vi "FlatToRichniswitch_grpc_ConfigureScanTriggerRequest.vi"(5 "OutputClusterType":T1, 11 "InputCluster":T3) -> (3 "OutputCluster":T1)   [LabVIEW 2021, in "NI Switch_client.lvlib"]
uses:
  NI Switch_client.lvlib
  niswitch_grpc_ConfigureScanTriggerRequest_trigger_input_enum/niswitch_grpc_ConfigureScanTriggerRequest_trigger_input_enum.lvclass
  niswitch_grpc_ConfigureScanTriggerRequest_scan_advanced_output_enum/niswitch_grpc_ConfigureScanTriggerRequest_scan_advanced_output_enum.lvclass
  nidevice_grpc_Session.ctl
  niswitch_grpc_ConfigureScanTriggerRequest.ctl
  niswitch_grpc_ScanAdvancedOutput.ctl
  niswitch_grpc_TriggerInput.ctl
  nidevice_grpc_Session_Flat.ctl
  niswitch_grpc_ConfigureScanTriggerRequest_Flat.ctl
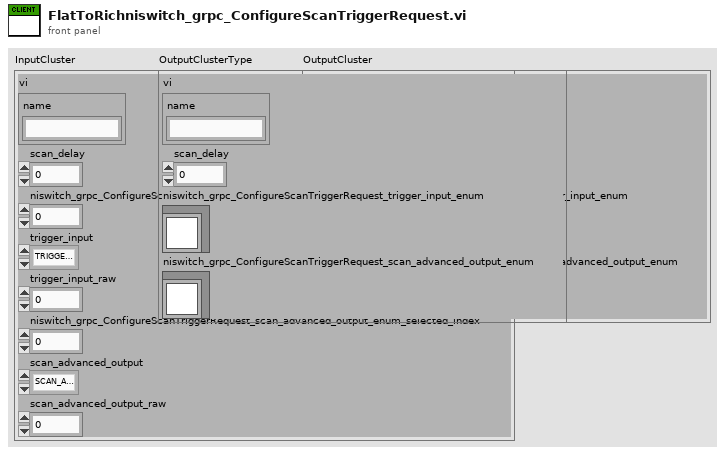
[diagram p1: front panel]
types:
  T1 = typedef "NI Switch_client.lvlib/niswitch_grpc_ConfigureScanTriggerRequest.ctl" = cluster{"vi":T2, "scan_delay":dbl, "niswitch_grpc_ConfigureScanTriggerRequest_trigger_input_enum":refnum<class "niswitch_grpc_ConfigureScanTriggerRequest_trigger_input_enum.lvclass">, "niswitch_grpc_ConfigureScanTriggerRequest_scan_advanced_output_enum":refnum<class "niswitch_grpc_ConfigureScanTriggerRequest_scan_advanced_output_enum.lvclass">}
  T2 = typedef "NI Switch_client.lvlib/nidevice_grpc_Session.ctl" = cluster{"name":string}
  T3 = typedef "NI Switch_client.lvlib/niswitch_grpc_ConfigureScanTriggerRequest_Flat.ctl" = cluster{"vi":T4, "scan_delay":dbl, "niswitch_grpc_ConfigureScanTriggerRequest_trigger_input_enum_selected_index":i32, "trigger_input":T5, "trigger_input_raw":i32, "niswitch_grpc_ConfigureScanTriggerRequest_scan_advanced_output_enum_selected_index":i32, "scan_advanced_output":T6, "scan_advanced_output_raw":i32}
  T4 = typedef "NI Switch_client.lvlib/nidevice_grpc_Session_Flat.ctl" = cluster{"name":string}
  T5 = typedef "NI Switch_client.lvlib/niswitch_grpc_TriggerInput.ctl" = enum32{"TRIGGER_INPUT_UNSPECIFIED", "TRIGGER_INPUT_NISWITCH_VAL_IMMEDIATE", "TRIGGER_INPUT_NISWITCH_VAL_EXTERNAL", "TRIGGER_INPUT_NISWITCH_VAL_SOFTWARE_TRIG", "TRIGGER_INPUT_NISWITCH_VAL_TTL0", "TRIGGER_INPUT_NISWITCH_VAL_TTL1", "TRIGGER_INPUT_NISWITCH_VAL_TTL2", "TRIGGER_INPUT_NISWITCH_VAL_TTL3", "TRIGGER_INPUT_NISWITCH_VAL_TTL4", "TRIGGER_INPUT_NISWITCH_VAL_TTL5", "TRIGGER_INPUT_NISWITCH_VAL_TTL6", "TRIGGER_INPUT_NISWITCH_VAL_TTL7", "TRIGGER_INPUT_NISWITCH_VAL_PXI_STAR", "TRIGGER_INPUT_NISWITCH_VAL_REARCONNECTOR", "TRIGGER_INPUT_NISWITCH_VAL_FRONTCONNECTOR", "TRIGGER_INPUT_NISWITCH_VAL_REARCONNECTOR_MODULE1", "TRIGGER_INPUT_NISWITCH_VAL_REARCONNECTOR_MODULE2", "TRIGGER_INPUT_NISWITCH_VAL_REARCONNECTOR_MODULE3", "TRIGGER_INPUT_NISWITCH_VAL_REARCONNECTOR_MODULE4", "TRIGGER_INPUT_NISWITCH_VAL_REARCONNECTOR_MODULE5", "TRIGGER_INPUT_NISWITCH_VAL_REARCONNECTOR_MODULE6", "TRIGGER_INPUT_NISWITCH_VAL_REARCONNECTOR_MODULE7", "TRIGGER_INPUT_NISWITCH_VAL_REARCONNECTOR_MODULE8", "TRIGGER_INPUT_NISWITCH_VAL_REARCONNECTOR_MODULE9", "TRIGGER_INPUT_NISWITCH_VAL_REARCONNECTOR_MODULE10", "TRIGGER_INPUT_NISWITCH_VAL_REARCONNECTOR_MODULE11", "TRIGGER_INPUT_NISWITCH_VAL_REARCONNECTOR_MODULE12", "TRIGGER_INPUT_NISWITCH_VAL_FRONTCONNECTOR_MODULE1", "TRIGGER_INPUT_NISWITCH_VAL_FRONTCONNECTOR_MODULE2", "TRIGGER_INPUT_NISWITCH_VAL_FRONTCONNECTOR_MODULE3", "TRIGGER_INPUT_NISWITCH_VAL_FRONTCONNECTOR_MODULE4", "TRIGGER_INPUT_NISWITCH_VAL_FRONTCONNECTOR_MODULE5", "TRIGGER_INPUT_NISWITCH_VAL_FRONTCONNECTOR_MODULE6", "TRIGGER_INPUT_NISWITCH_VAL_FRONTCONNECTOR_MODULE7", "TRIGGER_INPUT_NISWITCH_VAL_FRONTCONNECTOR_MODULE8", "TRIGGER_INPUT_NISWITCH_VAL_FRONTCONNECTOR_MODULE9", "TRIGGER_INPUT_NISWITCH_VAL_FRONTCONNECTOR_MODULE10", "TRIGGER_INPUT_NISWITCH_VAL_FRONTCONNECTOR_MODULE11", "TRIGGER_INPUT_NISWITCH_VAL_FRONTCONNECTOR_MODULE12"}
  T6 = typedef "NI Switch_client.lvlib/niswitch_grpc_ScanAdvancedOutput.ctl" = enum32{"SCAN_ADVANCED_OUTPUT_NISWITCH_VAL_NONE", "SCAN_ADVANCED_OUTPUT_NISWITCH_VAL_EXTERNAL", "SCAN_ADVANCED_OUTPUT_NISWITCH_VAL_TTL0", "SCAN_ADVANCED_OUTPUT_NISWITCH_VAL_TTL1", "SCAN_ADVANCED_OUTPUT_NISWITCH_VAL_TTL2", "SCAN_ADVANCED_OUTPUT_NISWITCH_VAL_TTL3", "SCAN_ADVANCED_OUTPUT_NISWITCH_VAL_TTL4", "SCAN_ADVANCED_OUTPUT_NISWITCH_VAL_TTL5", "SCAN_ADVANCED_OUTPUT_NISWITCH_VAL_TTL6", "SCAN_ADVANCED_OUTPUT_NISWITCH_VAL_TTL7", "SCAN_ADVANCED_OUTPUT_NISWITCH_VAL_PXI_STAR", "SCAN_ADVANCED_OUTPUT_NISWITCH_VAL_REARCONNECTOR", "SCAN_ADVANCED_OUTPUT_NISWITCH_VAL_FRONTCONNECTOR", "SCAN_ADVANCED_OUTPUT_NISWITCH_VAL_REARCONNECTOR_MODULE1", "SCAN_ADVANCED_OUTPUT_NISWITCH_VAL_REARCONNECTOR_MODULE2", "SCAN_ADVANCED_OUTPUT_NISWITCH_VAL_REARCONNECTOR_MODULE3", "SCAN_ADVANCED_OUTPUT_NISWITCH_VAL_REARCONNECTOR_MODULE4", "SCAN_ADVANCED_OUTPUT_NISWITCH_VAL_REARCONNECTOR_MODULE5", "SCAN_ADVANCED_OUTPUT_NISWITCH_VAL_REARCONNECTOR_MODULE6", "SCAN_ADVANCED_OUTPUT_NISWITCH_VAL_REARCONNECTOR_MODULE7", "SCAN_ADVANCED_OUTPUT_NISWITCH_VAL_REARCONNECTOR_MODULE8", "SCAN_ADVANCED_OUTPUT_NISWITCH_VAL_REARCONNECTOR_MODULE9", "SCAN_ADVANCED_OUTPUT_NISWITCH_VAL_REARCONNECTOR_MODULE10", "SCAN_ADVANCED_OUTPUT_NISWITCH_VAL_REARCONNECTOR_MODULE11", "SCAN_ADVANCED_OUTPUT_NISWITCH_VAL_REARCONNECTOR_MODULE12", "SCAN_ADVANCED_OUTPUT_NISWITCH_VAL_FRONTCONNECTOR_MODULE1", "SCAN_ADVANCED_OUTPUT_NISWITCH_VAL_FRONTCONNECTOR_MODULE2", "SCAN_ADVANCED_OUTPUT_NISWITCH_VAL_FRONTCONNECTOR_MODULE3", "SCAN_ADVANCED_OUTPUT_NISWITCH_VAL_FRONTCONNECTOR_MODULE4", "SCAN_ADVANCED_OUTPUT_NISWITCH_VAL_FRONTCONNECTOR_MODULE5", "SCAN_ADVANCED_OUTPUT_NISWITCH_VAL_FRONTCONNECTOR_MODULE6", "SCAN_ADVANCED_OUTPUT_NISWITCH_VAL_FRONTCONNECTOR_MODULE7", "SCAN_ADVANCED_OUTPUT_NISWITCH_VAL_FRONTCONNECTOR_MODULE8", "SCAN_ADVANCED_OUTPUT_NISWITCH_VAL_FRONTCONNECTOR_MODULE9", "SCAN_ADVANCED_OUTPUT_NISWITCH_VAL_FRONTCONNECTOR_MODULE10", "SCAN_ADVANCED_OUTPUT_NISWITCH_VAL_FRONTCONNECTOR_MODULE11", "SCAN_ADVANCED_OUTPUT_NISWITCH_VAL_FRONTCONNECTOR_MODULE12"}
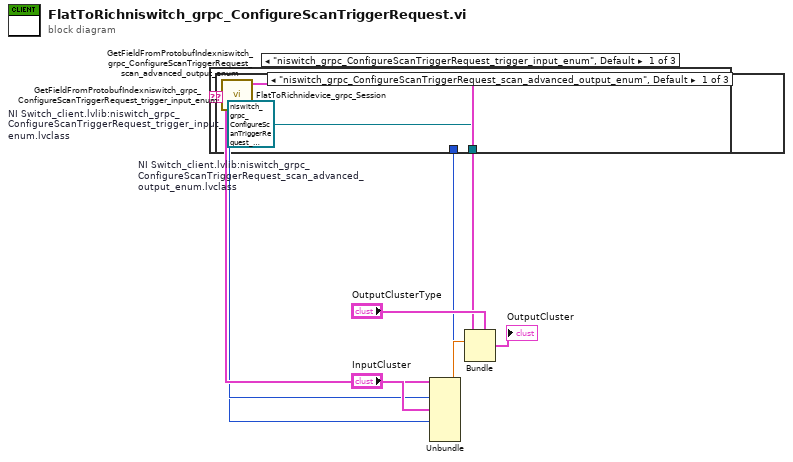
[diagram p0: block diagram]
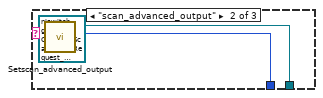
[diagram p2: hidden frame]
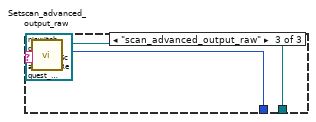
[diagram p3: hidden frame]
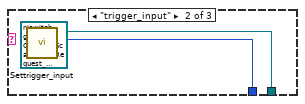
[diagram p4: hidden frame]
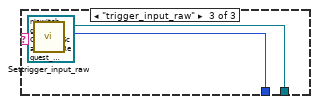
[diagram p5: hidden frame]
diagram:
  n1 = Unbundle "Unbundle"("InputCluster") -> ("vi"=w13:T4, "scan_delay"=w11:dbl, "niswitch_grpc_ConfigureScanTriggerRequest_trigger_input_enum_selected_index"=w10:i32, "trigger_input"=w7:T5, "trigger_input_raw"=w6:i32, "niswitch_grpc_ConfigureScanTriggerRequest_scan_advanced_output_enum_selected_index"=w5:i32, "scan_advanced_output"=w2:T6, "scan_advanced_output_raw"=w1:i32)
  n2 = call "GetFieldFromProtobufIndexniswitch_grpc_ConfigureScanTriggerRequest_scan_advanced_output_enum.vi"("protobuf index"=w5) -> ("oneof field name"=w4:string)
  n3 = case "niswitch_grpc_ConfigureScanTriggerRequest_scan_advanced_output_enum" shown="\"niswitch_grpc_ConfigureScanTriggerRequest_scan_advanced_output_enum\", Default" w4 {
    tunnel: [w17 w19 w22] -> w3
    tunnel: w2 -> [_ w20 _]
    tunnel: w1 -> [_ _ w23]
    frame "niswitch_grpc_ConfigureScanTriggerRequest_scan_advanced_output_enum", Default {
      w17 = refnum<class "niswitch_grpc_ConfigureScanTriggerRequest_scan_advanced_output_enum.lvclass"> refnum  # NI Switch_client.lvlib:niswitch_grpc_ConfigureScanTriggerRequest_scan_advanced_output_enum.lvclass
    }
    frame "scan_advanced_output" {
      n4 = call "Setscan_advanced_output.vi"("Set_Val"=w20, "OneOfTemplate in"=refnum<class "niswitch_grpc_ConfigureScanTriggerRequest_scan_advanced_output_enum.lvclass"> refnum) -> ("OneOfTemplate out"=w19:refnum<class "niswitch_grpc_ConfigureScanTriggerRequest_scan_advanced_output_enum.lvclass">)  [unwired: 8 in, 1 out]
    }
    frame "scan_advanced_output_raw" {
      n5 = call "Setscan_advanced_output_raw.vi"("Set_Val"=w23, "OneOfTemplate in"=refnum<class "niswitch_grpc_ConfigureScanTriggerRequest_scan_advanced_output_enum.lvclass"> refnum) -> ("OneOfTemplate out"=w22:refnum<class "niswitch_grpc_ConfigureScanTriggerRequest_scan_advanced_output_enum.lvclass">)  [unwired: 8 in, 1 out]
    }
  }
  n6 = call "GetFieldFromProtobufIndexniswitch_grpc_ConfigureScanTriggerRequest_trigger_input_enum.vi"("protobuf index"=w10) -> ("oneof field name"=w9:string)
  n7 = case "niswitch_grpc_ConfigureScanTriggerRequest_trigger_input_enum" shown="\"niswitch_grpc_ConfigureScanTriggerRequest_trigger_input_enum\", Default" w9 {
    tunnel: [w24 w26 w29] -> w8
    tunnel: w7 -> [_ w27 _]
    tunnel: w6 -> [_ _ w30]
    frame "niswitch_grpc_ConfigureScanTriggerRequest_trigger_input_enum", Default {
      w24 = refnum<class "niswitch_grpc_ConfigureScanTriggerRequest_trigger_input_enum.lvclass"> refnum  # NI Switch_client.lvlib:niswitch_grpc_ConfigureScanTriggerRequest_trigger_input_enum.lvclass
    }
    frame "trigger_input" {
      n8 = call "Settrigger_input.vi"("Set_Val"=w27, "OneOfTemplate in"=refnum<class "niswitch_grpc_ConfigureScanTriggerRequest_trigger_input_enum.lvclass"> refnum) -> ("OneOfTemplate out"=w26:refnum<class "niswitch_grpc_ConfigureScanTriggerRequest_trigger_input_enum.lvclass">)  [unwired: 8 in, 1 out]
    }
    frame "trigger_input_raw" {
      n9 = call "Settrigger_input_raw.vi"("Set_Val"=w30, "OneOfTemplate in"=refnum<class "niswitch_grpc_ConfigureScanTriggerRequest_trigger_input_enum.lvclass"> refnum) -> ("OneOfTemplate out"=w29:refnum<class "niswitch_grpc_ConfigureScanTriggerRequest_trigger_input_enum.lvclass">)  [unwired: 8 in, 1 out]
    }
  }
  n10 = call "FlatToRichnidevice_grpc_Session.vi"("InputCluster"=w13) -> ("OutputCluster"=w12:T2)  [unwired: 10 in]
  n11 = Bundle "Bundle"(cluster="OutputClusterType", "vi"=w12, "scan_delay"=w11, "niswitch_grpc_ConfigureScanTriggerRequest_trigger_input_enum"=w8, "niswitch_grpc_ConfigureScanTriggerRequest_scan_advanced_output_enum"=w3) -> (→"OutputCluster":T1)
